vi "Update History Dst Q.vi"(8 "error in (no error)":errorcluster, 10 "Update History Dst Q Data cluster":T1, 11 "Motions in":refnum<class "Motions.lvclass">) -> (0 "error out":errorcluster, 3 "Motions out":refnum<class "Motions.lvclass">)   [LabVIEW 2016, in "Hardware.lvlib" / "Motions.lvlib" / "Motions.lvclass"]
uses:
  <userlib>/Common Components/Hardware/Abstract System/Motions/Motions/Motions.lvclass
  <userlib>/Common Components/Hardware/Abstract System/Motions/Motions/Data_Update History Dst Q.ctl
  <userlib>/Common Components/Hardware/Abstract System/Motions/Motions/Motions.lvclass/Motions.ctl
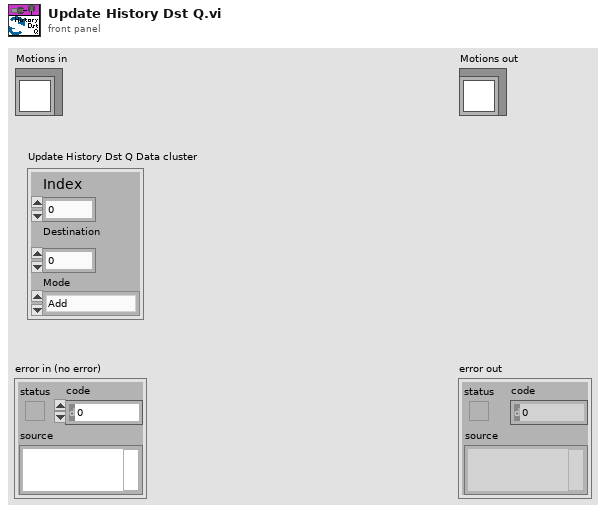
[diagram p1: front panel]
types:
  T1 = typedef "Hardware.lvlib/Motions.lvlib/Motions.lvclass/Data_Update History Dst Q.ctl" = cluster{"Index":i32, "Destination":dbl, "Mode":enum16{"Add", "Replace"}}
  T2 = typedef "Hardware.lvlib/Motions.lvlib/Motions.lvclass/Motor States.ctl" = cluster{"Connected":bool, "Enabled":bool, "Moving Status":bool, "Soft Moving Status":bool, "Current Pos":dbl, "Target Pos":dbl, "Moving Dir (-1, 0, 1)":i32, "Error Status":bool, "Hard Limit+":bool, "Hard Limit-":bool, "Soft Limit+":bool, "Soft Limit-":bool, "History Dst Stack":refnum<queue>, "Motion Status":bool, "Motion TriggerAction Obj":refnum<class "TriggerAction.lvclass">}
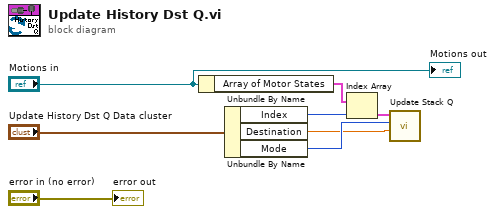
[diagram p0: block diagram]
diagram:
  n1 = Unbundle By Name("Motions in") -> ("Array of Motor States"=w5:T2[])
  n2 = Unbundle By Name("Update History Dst Q Data cluster") -> ("Index"=w4:i32, "Destination"=w1:dbl, "Mode"=w2:enum16{"Add", "Replace"})
  n3 = Index Array(array=w5, index=w4) -> (element=w3:T2)
  n4 = call <userlib>:"Update Stack Q.vi"("Destination"=w1, "Mode"=w2, "Motor States"=w3) -> ()  [unwired: 9 in]
  "error out" <- "error in (no error)"
  "Motions out" <- "Motions in"
